vi "Excel Error Helper.vi"(0 "error in 1":errorcluster, 7 "message":string=" (please make sure that Microsoft Excel is installed on your system)", 11 "error in 2":errorcluster) -> (15 "error out":errorcluster)   [LabVIEW 2017, in "NI_ReportGenerationToolkit.lvlib"]
uses:
  <vilib>/addons/_office/NI_ReportGenerationToolkit.lvlib
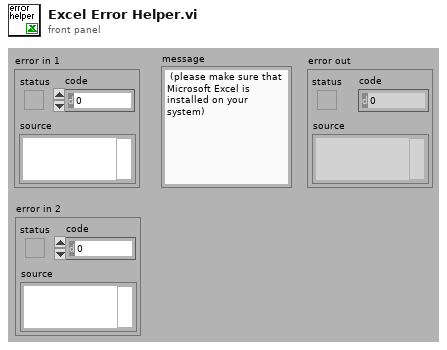
[diagram p1: front panel]
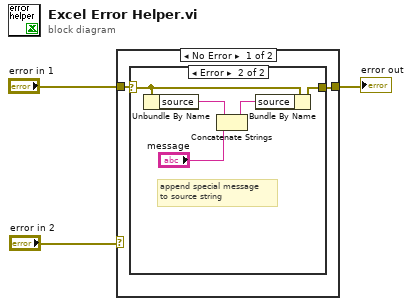
[diagram p0: block diagram]
diagram:
  n1 = case shown="No Error" "error in 2" {
    tunnel: "error in 1" -> [w5 w12]
    tunnel: [w4 w12] -> w1
    frame No Error {
      n2 = case shown="Error" w5 {
        selector: w5 -> [w6 w11]
        tunnel: [w6 w10] -> w4
        frame No Error {
        }
        frame Error {
          # "append special message\nto source string"
          n3 = Unbundle By Name(w11) -> ("source"=w9:string)
          n4 = Concatenate Strings(w9, "message") -> (w8:string)
          n5 = Bundle By Name(cluster=w11, "source"=w8) -> (w10:errorcluster)
        }
      }
    }
    frame Error {
    }
  }
  "error out" <- w1
